vi "GETPORTSTATUS.vi"(8 "error in (no error)":errorcluster, 10 "Port to read":dbl, 11 "Arduino in":refnum<class "Arduino.lvclass">) -> (0 "error out":errorcluster, 3 "Arduino out":refnum<class "Arduino.lvclass">)   [LabVIEW 2019, in "Arduino.lvclass"]
uses:
  Arduino.lvclass
  Arduino.lvclass/Arduino.ctl
  41c01e4d-bb9d-4a94-b4d1-ad617550b47b.vi
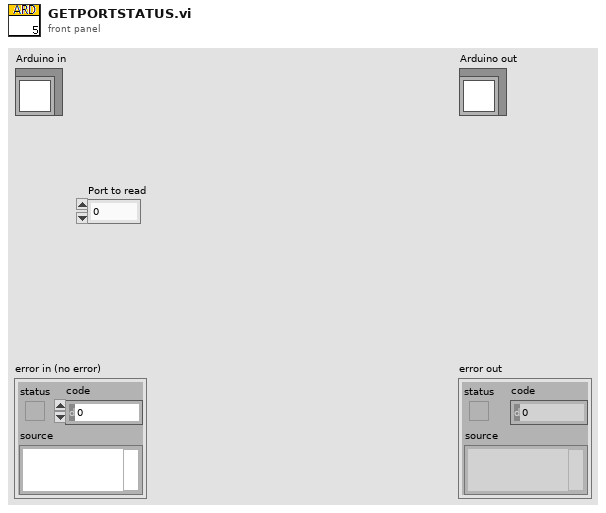
[diagram p1: front panel]
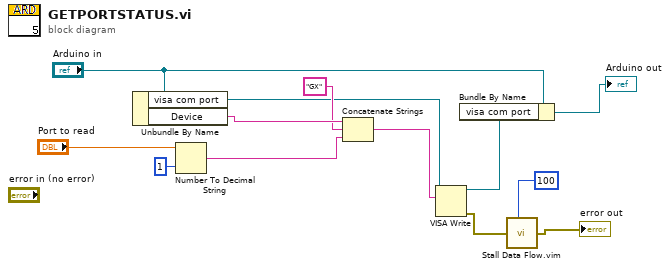
[diagram p0: block diagram]
diagram:
  n1 = Unbundle By Name("Arduino in") -> ("visa com port"=w7:refnum<visa-resource-name>, "Device"=w11:string)
  n2 = Number To Decimal String(number="Port to read", width (-)=i16 1) -> (decimal integer string=w9:string)
  n3 = Concatenate Strings(w11, "GX" ("string"), w9) -> (w8:string)
  n4 = VISA Write(VISA resource name=w7, write buffer=w8) -> (VISA resource name out=w1:refnum<visa-resource-name>, error out=w6:errorcluster)  [unwired: 1 in, 1 out]
  n5 = Bundle By Name(cluster="Arduino in", "visa com port"=w1) -> (→"Arduino out":refnum<class "Arduino.lvclass">)
  n6 = call "Stall Data Flow.vim"("value in"=w6, "milliseconds to wait"=u32 100) -> ("value out"=→"error out":errorcluster)  [unwired: 1 out]
